vi "locate tag of unknown type.vi"(8 "error in":errorcluster, 10 "name":string, 11 "data dictionary in":refnum<class "data dictionary.lvclass">) -> (0 "error out":errorcluster, 1 "data type":T1, 2 "index":i32, 3 "data dictionary out":refnum<class "data dictionary.lvclass">)   [LabVIEW 2013, in "tag bus.lvlib" / "data dictionary.lvclass"]
doc: "Performs a search through every data type in the dictionary to find the type and index of a tag."
uses:
  data dictionary.lvclass
  tag/Data Type.ctl
  tag/tag descriptor.lvclass
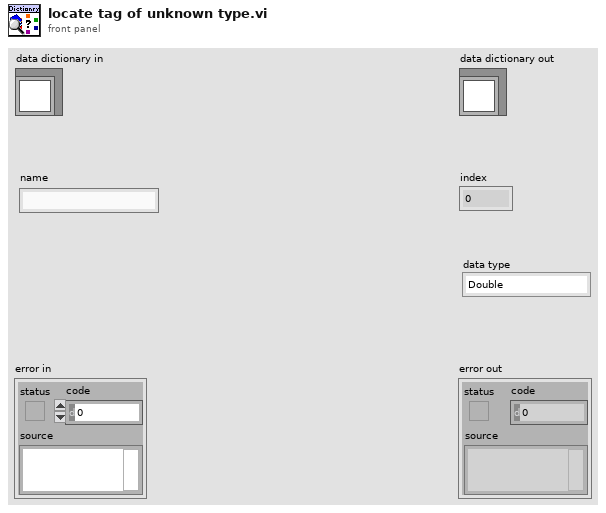
[diagram p1: front panel]
types:
  T1 = typedef "tag bus.lvlib/tag descriptor.lvclass/Data Type.ctl" = enum16{"Double", "Single", "I64", "I32", "I16", "I8", "U64", "U32", "U16", "U8", "Boolean", "String", "Array of Double", "Array of Single", "Array of I64", "Array of I32", "Array of I16", "Array of I8", "Array of U64", "Array of U32", "Array of U16", "Array of U8", "Array of Boolean", "Array of String"}
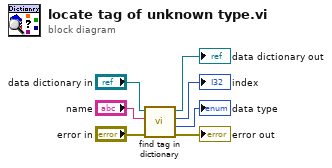
[diagram p0: block diagram]
diagram:
  n1 = call "find tag in dictionary.vi"("error in"="error in", "name"="name", "data dictionary in"="data dictionary in") -> ("error out"=→"error out":errorcluster, "actual data type"=→"data type":T1, "index"=→"index":i32, "data dictionary out"=→"data dictionary out":refnum<class "data dictionary.lvclass">)  [unwired: 5 in]
